vi "Test DAQmx Synthesizer.vi"() -> ()   [LabVIEW 2019]
uses:
  DAQmx Synthesizer Configuration.ctl
  DAQmx Synthesizer.lvclass
  DAQmx Synthesizer.lvclass/DAQmx Synthesizer.ctl
  Write DAQmx Device Name.vi
  Read Waveforms.vi
panel:
  in  "Stop Button":bool
  out "Waveform Graph":waveform(dbl)[](graph)
  in  "DAQmx Device Name 2":tag
  out "Finished":bool
  in  "User Configuration":T1={"Ranges"=[10.0], "Channel names"=["Bdot"], "Output channels"="0", "File Path Control"=path "", "Offset"=1.0, "Scale"=0.5} {"Ranges" format="%#_6pV"}
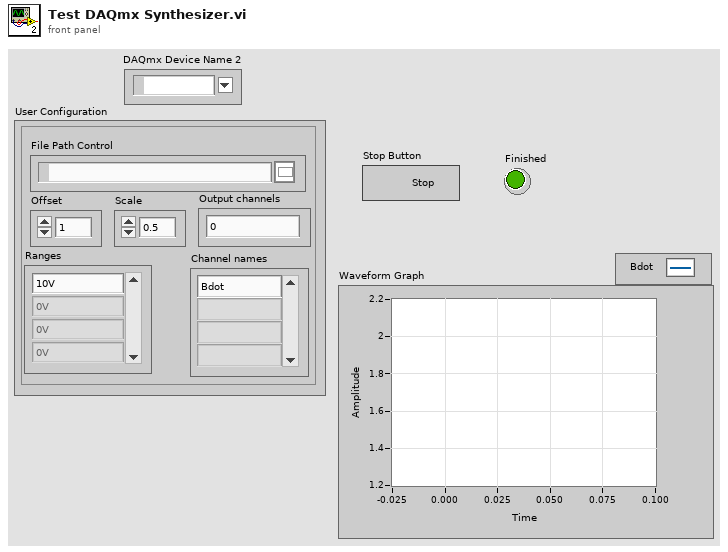
[diagram p1: front panel]
types:
  T1 = typedef "DAQmx Synthesizer Configuration.ctl" = cluster{"Ranges":dbl[], "Channel names":string[], "Output channels":string, "File Path Control":path, "Offset":dbl, "Scale":dbl}
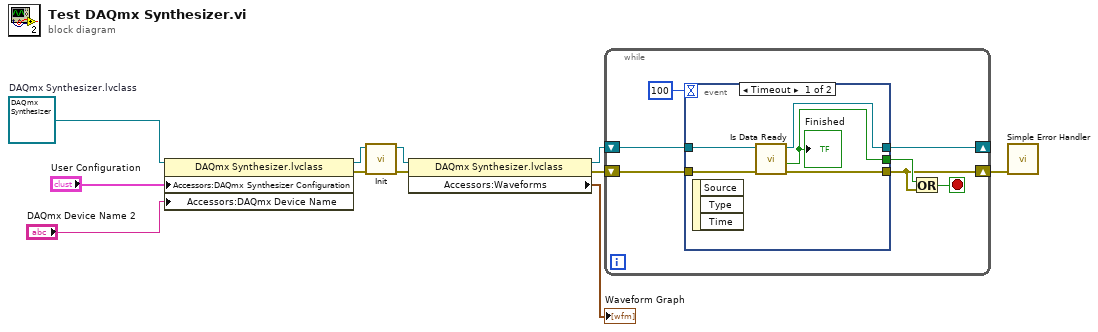
[diagram p0: block diagram]
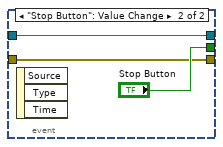
[diagram p2: hidden frame]
diagram:
  w11 = refnum<class "DAQmx Synthesizer.lvclass"> refnum  # DAQmx Synthesizer.lvclass
  n1 = property class="DAQmx Synthesizer.lvclass"(reference=w11, "Accessors:DAQmx Synthesizer Configuration"="User Configuration", "Accessors:DAQmx Device Name"="DAQmx Device Name 2") -> (reference out=w10:refnum<class "DAQmx Synthesizer.lvclass">, error out=w9:errorcluster)  [unwired: 1 in]
  n2 = call-dynamic "Init.vi"("error in (no error)"=w9, "Instrument Driver in"=w10) -> ("error out"=w8:errorcluster, "Instrument Driver out"=w5:refnum<class "DAQmx Synthesizer.lvclass">)  [unwired: 6 in, 2 out]
  n3 = property class="DAQmx Synthesizer.lvclass"(reference=w5, error in=w8) -> (reference out=w3:refnum<class "DAQmx Synthesizer.lvclass">, error out=w2:errorcluster, "Accessors:Waveforms"=→"Waveform Graph":waveform(dbl)[])
  n4 = while {
    shift-right: [w15] -> _
    shift-left: w3 -> [w17]
    shift-right: [w12] -> w1
    shift-left: w2 -> [w16]
    stop <- w14 stop-if-true
    n5 = event shown="[0] Timeout" {
      selector: _ -> [_ _]
      dyn-events: _ -> [_ _]
      timeout: 100 -> [_ _]
      tunnel: [w19 "Stop Button"] -> w13
      tunnel: w17 -> [w23 w25]
      tunnel: w16 -> [w22 w24]
      tunnel: [w21 w24] -> w12
      tunnel: [w20 w25] -> w15
      event Timeout {
        n6 = event-data() -> ()  [unwired: 1 in, 3 out]
        n7 = call-dynamic "Is Data Ready.vi"("error in (no error)"=w22, "DAQmx Digitizer in"=w23) -> ("error out"=w21:errorcluster, "Data ready"=w19:bool, "DAQmx Digitizer out"=w20:refnum<class "DAQmx Synthesizer.lvclass">)  [unwired: 6 in, 1 out]
        "Finished" <- w19
      }
      event "Stop Button": Value Change {
        n8 = event-data() -> ()  [unwired: 1 in, 3 out]
      }
    }
    n9 = Or(x=w13, y=w12) -> (x .or. y?=w14:bool)
  }
  n10 = call <vilib>:"Simple Error Handler.vi"("error in (no error)"=w1) -> ()  [unwired: 4 in, 5 out]
